vi "Get value.vi"(0 "Stack in":refnum<class "Stack.lvclass">, 11 "error in (no error)":errorcluster) -> (3 "PUT Settings":T1, 4 "Stack out":refnum<class "Stack.lvclass">, 6 "Resolution Geometry":string, 10 "Assembly Settings":T1, 13 "Is real run":bool, 14 "Component Settings":T1, 15 "error out":errorcluster)   [LabVIEW 2021, in "Stack.lvclass"]
uses:
  Stack.lvclass
  Stack.lvclass/Stack.ctl
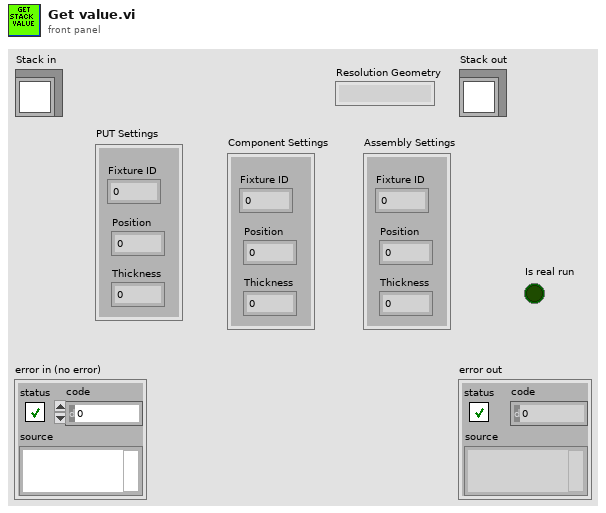
[diagram p1: front panel]
types:
  T1 = cluster{"Fixture ID":dbl, "Position":dbl, "Thickness":dbl}
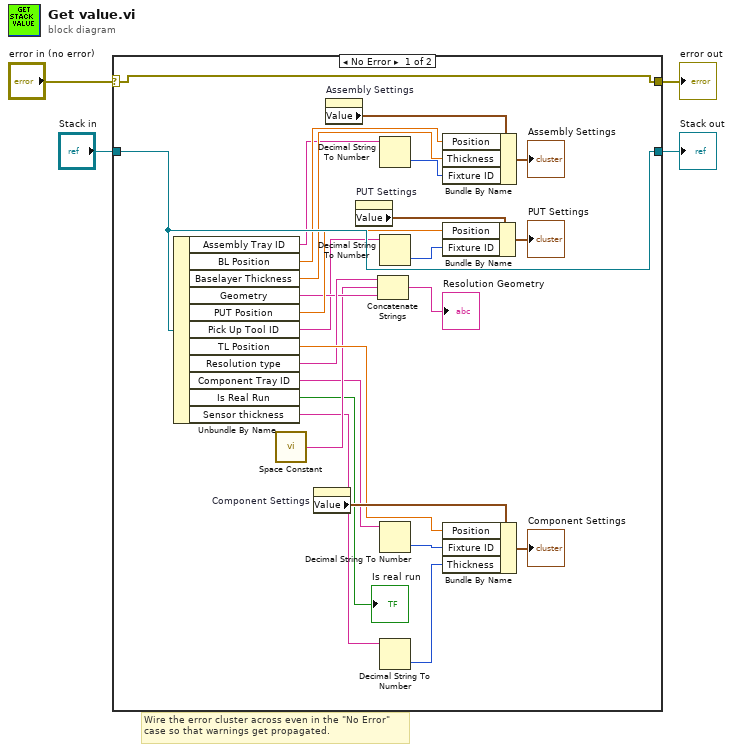
[diagram p0: block diagram]
diagram:
  # "Wire the error cluster across even in the \"No Error\"\ncase so that warnings get propagated."
  n1 = case shown="No Error" "error in (no error)" {
    selector: "error in (no error)" -> [w29 w31]
    tunnel: [w29 w31] -> w3
    tunnel: [w28 w30] -> w1
    tunnel: "Stack in" -> [w28 w30]
    frame No Error {
      n2 = Unbundle By Name(w28) -> ("Assembly Tray ID"=w13:string, "BL Position"=w24:dbl, "Baselayer Thickness"=w25:dbl, "Geometry"=w16:string, "PUT Position"=w19:dbl, "Pick Up Tool ID"=w9:string, "TL Position"=w18:dbl, "Resolution type"=w17:string, "Component Tray ID"=w12:string, "Is Real Run"=→"Is real run":bool, "Sensor thickness"=w6:string)
      n3 = call <vilib>:"Space Constant.vi"() -> ("String"=w14:string)
      n4 = property on="Component Settings" class="Clust (strict)"() -> ("Value"=w23:T1)  [unwired: 2 in, 2 out]
      n5 = property on="Assembly Settings" class="Clust (strict)"() -> ("Value"=w26:T1)  [unwired: 2 in, 2 out]
      n6 = property on="PUT Settings" class="Clust (strict)"() -> ("Value"=w21:T1)  [unwired: 2 in, 2 out]
      n7 = Concatenate Strings(w17, w14, w16) -> (→"Resolution Geometry":string)
      n8 = Decimal String To Number(string=w13) -> (number=w8:i32)  [unwired: 2 in, 1 out]
      n9 = Decimal String To Number(string=w9) -> (number=w10:i32)  [unwired: 2 in, 1 out]
      n10 = Decimal String To Number(string=w12) -> (number=w11:i32)  [unwired: 2 in, 1 out]
      n11 = Decimal String To Number(string=w6) -> (number=w5:i32)  [unwired: 2 in, 1 out]
      n12 = Bundle By Name(cluster=w26, "Position"=w24, "Thickness"=w25, "Fixture ID"=w8) -> (→"Assembly Settings":T1)
      n13 = Bundle By Name(cluster=w21, "Position"=w19, "Fixture ID"=w10) -> (→"PUT Settings":T1)
      n14 = Bundle By Name(cluster=w23, "Position"=w18, "Fixture ID"=w11, "Thickness"=w5) -> (→"Component Settings":T1)
    }
    frame Error {
    }
  }
  "error out" <- w3
  "Stack out" <- w1
